vi "interfaz para quiz1 (1).vi"() -> ()   [LabVIEW 2020]
panel:
  in  "stop":bool
  out "Led 3":bool
  out "Led 2":bool
  out "Led 1":bool
  in  "Pulsador 3":bool
  in  "Pulsador 2":bool
  in  "Pulsador 1":bool
  out "tiempo(ms)":i32=1000
  out "Contador":i32
  in  "Insertar trama":string
  out "RESPUESTA":string="\n      \n           "
  in  "Ingreso de comandos":string
  in  "?":bool
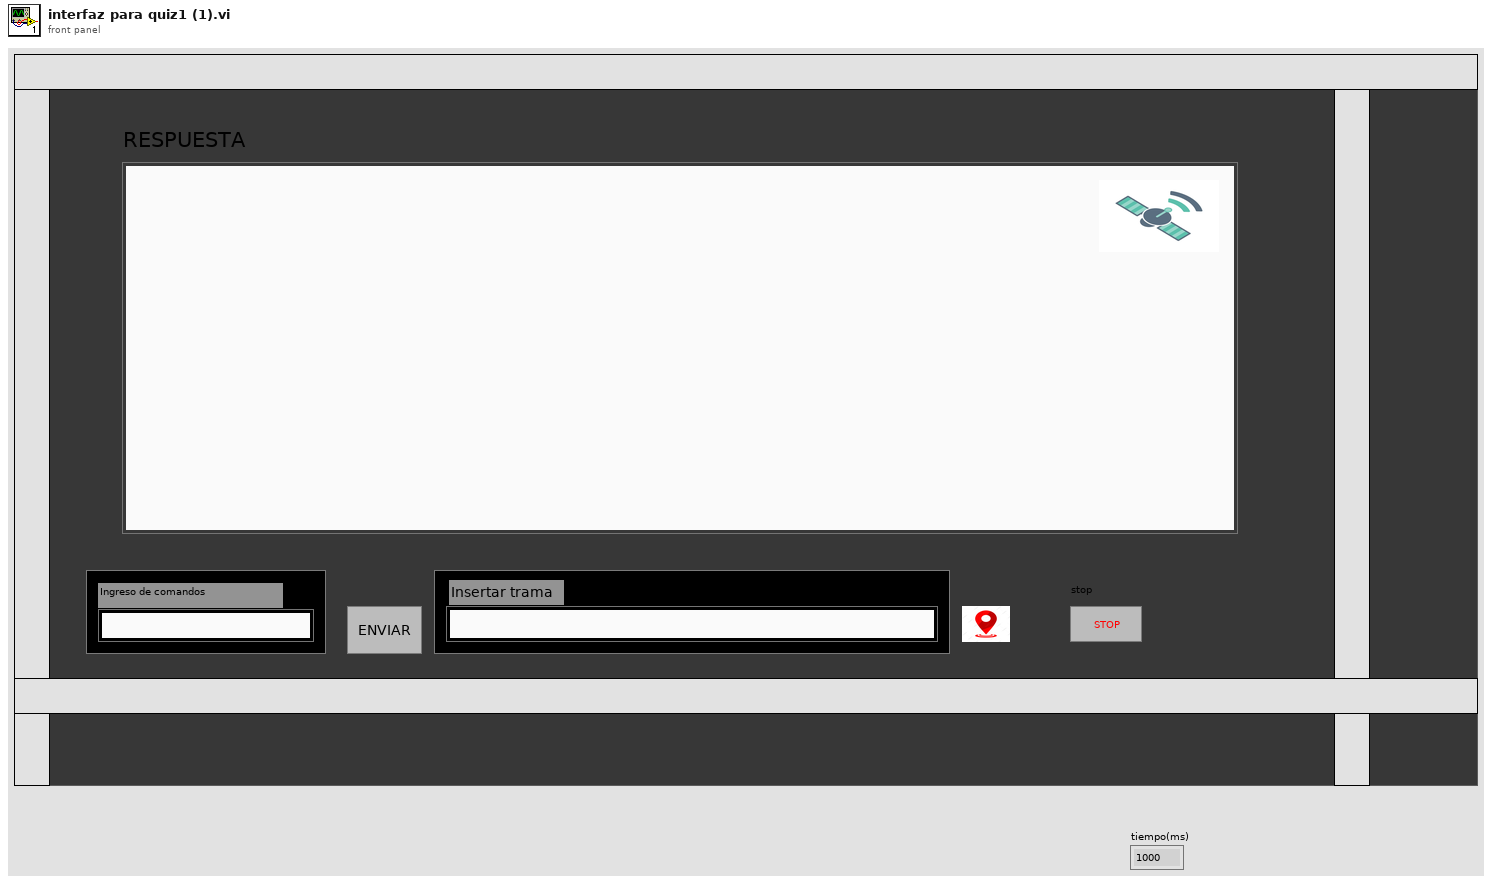
[diagram p1: front panel]
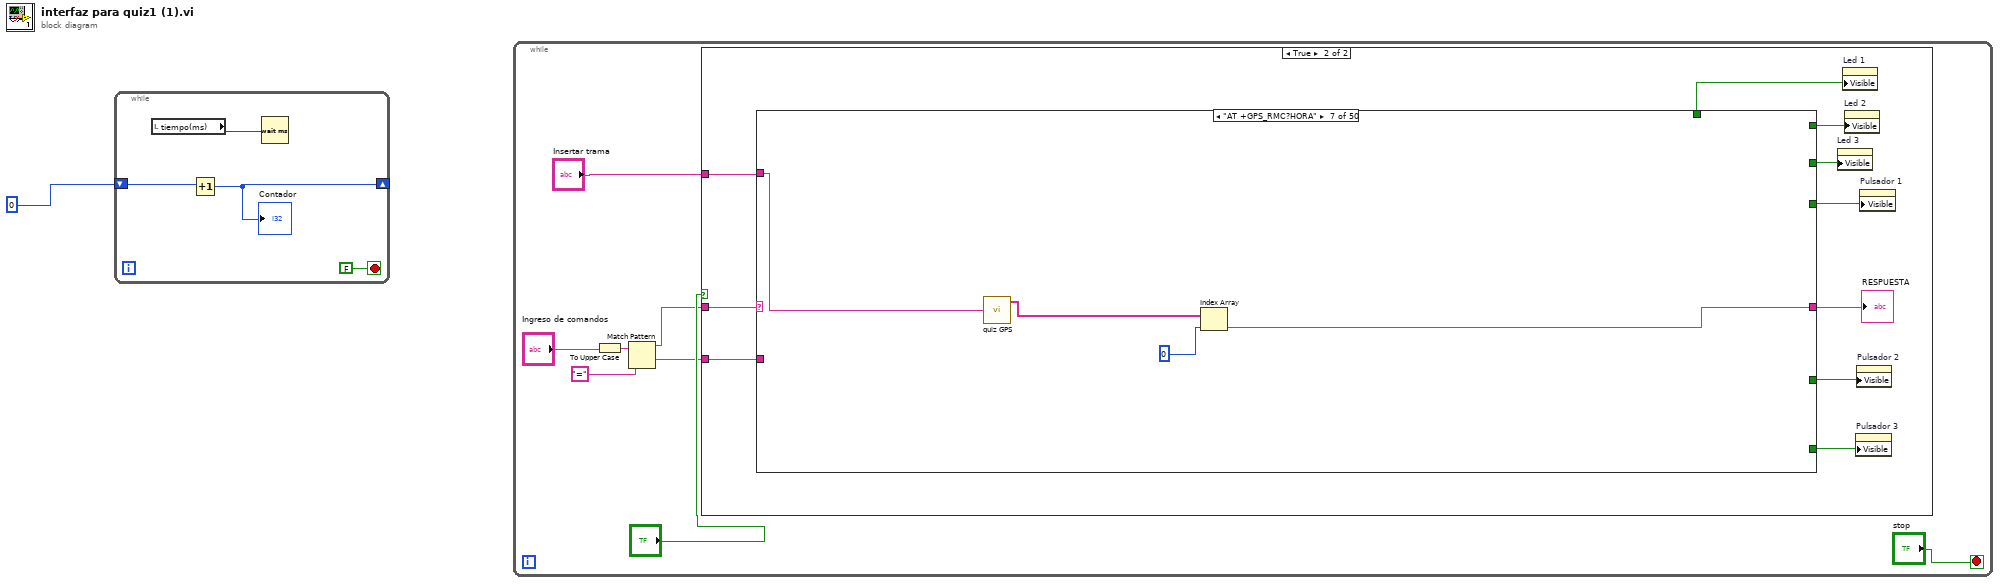
[diagram p0: block diagram]
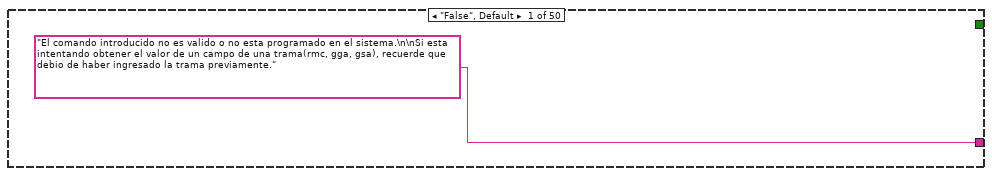
[diagram p3: hidden frame]
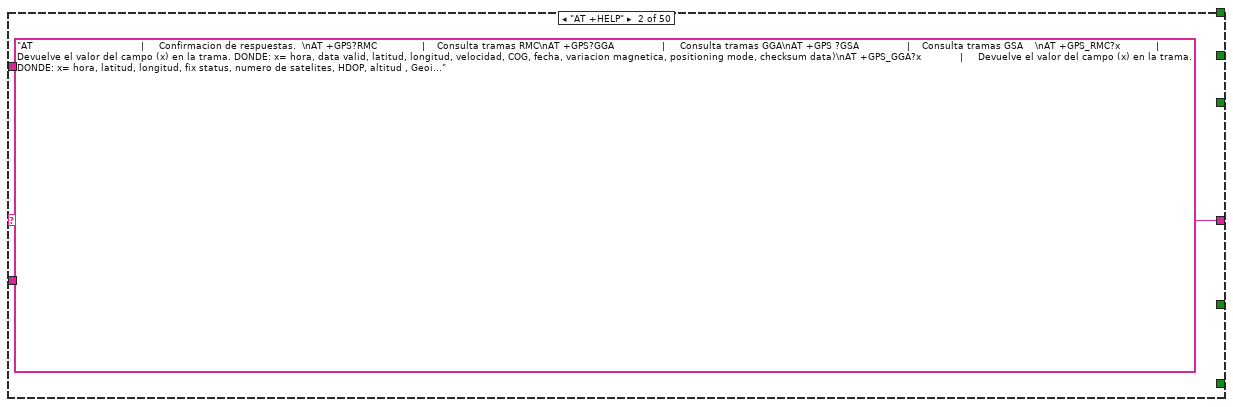
[diagram p4: hidden frame]
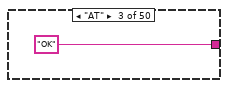
[diagram p5: hidden frame]
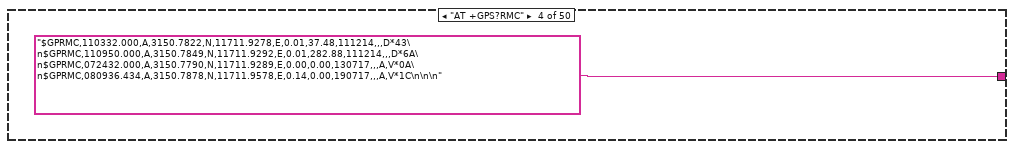
[diagram p6: hidden frame]
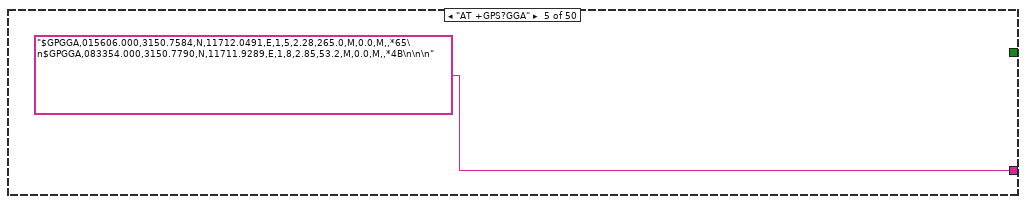
[diagram p7: hidden frame]
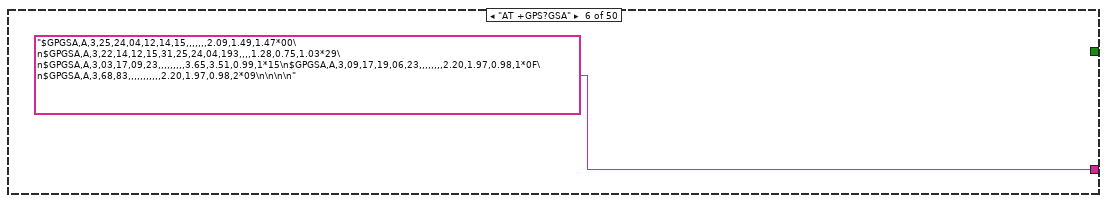
[diagram p8: hidden frame]
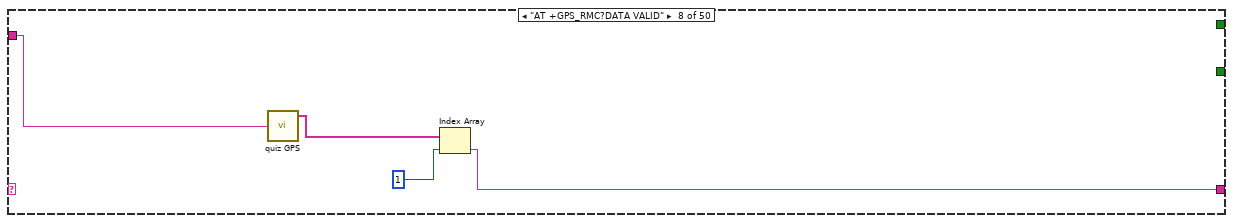
[diagram p9: hidden frame]
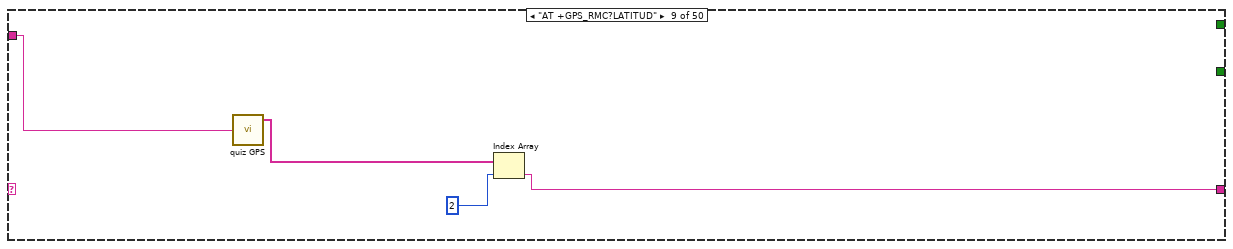
[diagram p10: hidden frame]
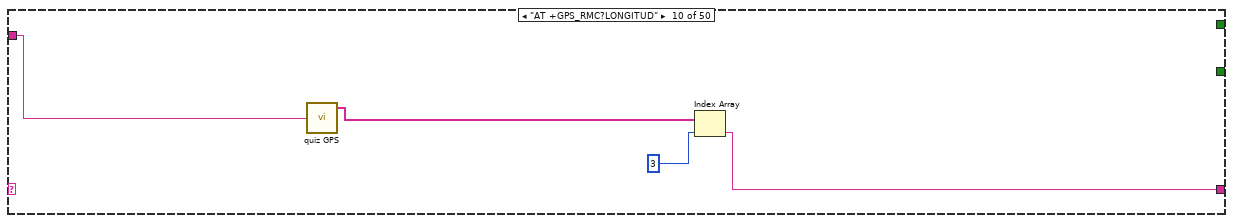
[diagram p11: hidden frame]
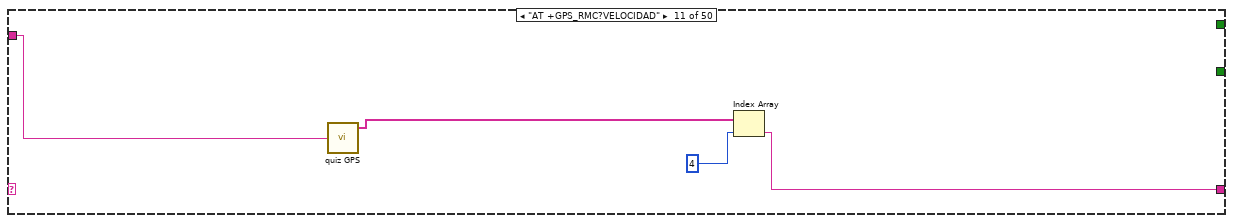
[diagram p12: hidden frame]
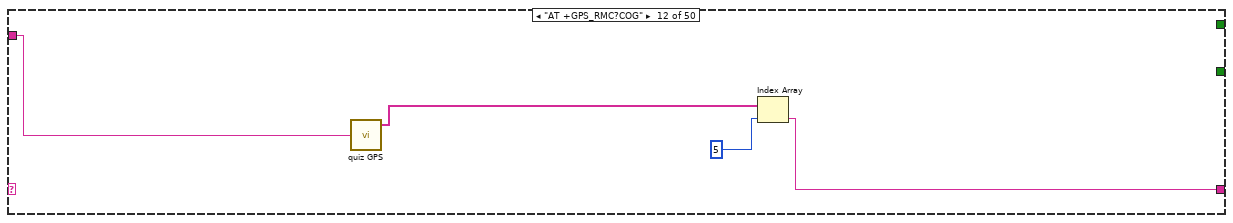
[diagram p13: hidden frame]
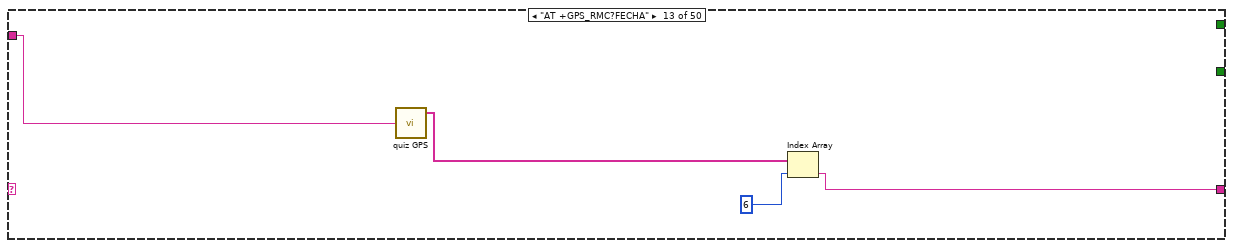
[diagram p14: hidden frame]
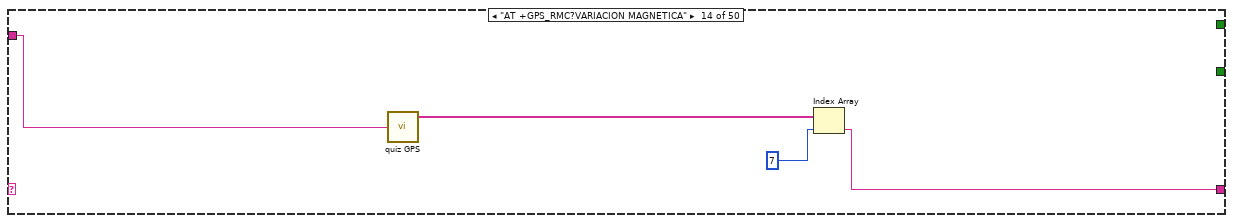
[diagram p15: hidden frame]
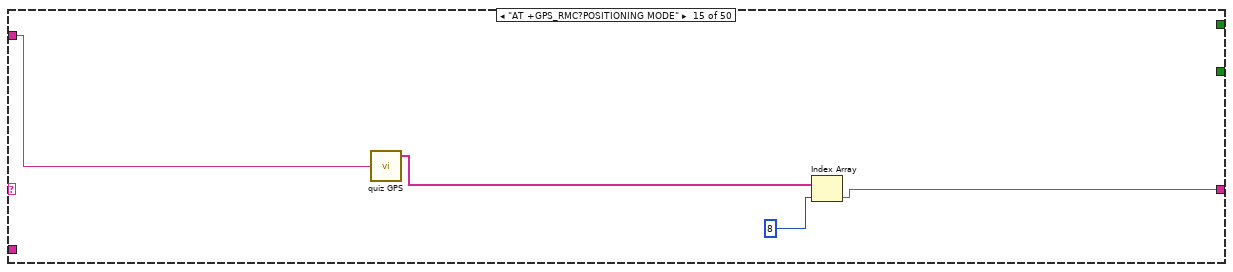
[diagram p16: hidden frame]
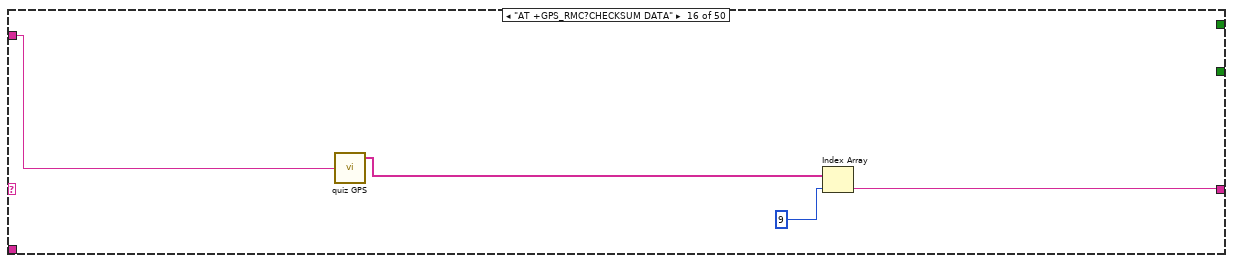
[diagram p17: hidden frame]
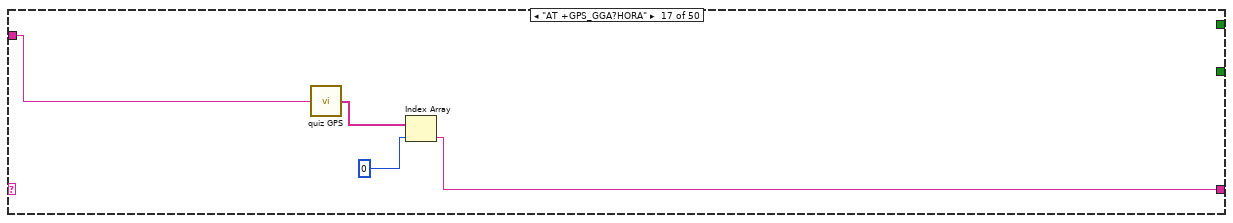
[diagram p18: hidden frame]
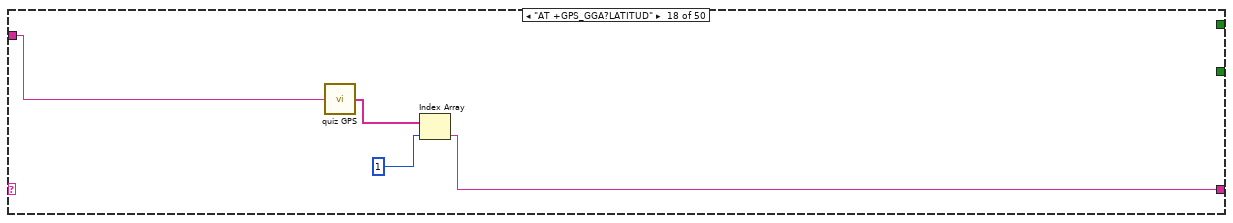
[diagram p19: hidden frame]
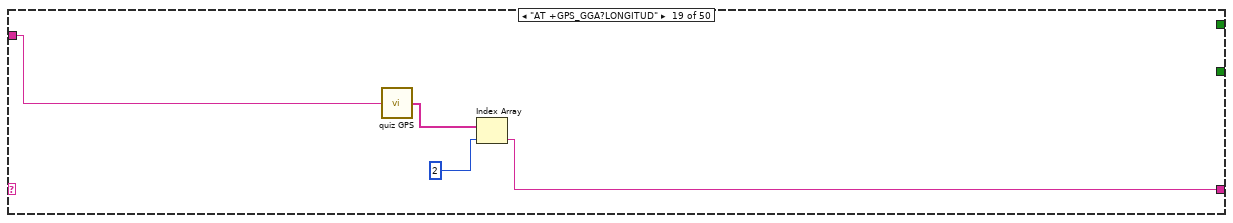
[diagram p20: hidden frame]
diagram:
  n1 = while {
    shift-right: [w2] -> _
    shift-left: 0 -> [w5]
    stop <- FALSE stop-if-true
    n2 = local read "tiempo(ms)"() -> (w3:i32)
    n3 = Increment(x=w5) -> (x+1=w2:i32)
    "Contador" <- w2
    n4 = Wait (ms)(milliseconds to wait=w3) -> ()  [unwired: 1 out]
  }
  n5 = while {
    stop <- "stop" stop-if-true
    n6 = To Upper Case(1:"Ingreso de comandos") -> (0:w10:string)
    n7 = Match Pattern(string=w10, regular expression="=") -> (before substring=w8:string, after substring=w7:string)  [unwired: 1 in, 2 out]
    n8 = case shown="True" "?" {
      tunnel: "Insertar trama" -> [_ w22]
      tunnel: w8 -> [_ w18]
      tunnel: w7 -> [_ w17]
      frame False {
      }
      frame True {
        n9 = case shown="\"AT +GPS_RMC?HORA\"" w18 {
          tunnel: ["El comando introducido no es valido o no esta programado en el sistema.\n\nSi esta intentando obtener el valor de un campo de una trama(rmc, gga, gsa), recuerde que debio de haber ingresado la trama previamente." "AT                                    |     Confirmacion de respuestas.  \nAT +GPS?RMC               |    Consulta tramas RMC\nAT +GPS?GGA                |     Consulta tramas GGA\nAT +GPS ?GSA                |    Consulta tramas GSA    \nAT +GPS_RMC?x            |     Devuelve el valor del campo (x) en la trama. DONDE: x= hora, data valid, latitud, longitud, velocidad, COG, fecha, variacion magnetica, positioning mode, checksum data)\nAT +GPS_GGA?x             |     Devuelve el valor del campo (x) en la trama. DONDE: x= hora, latitud, longitud, fix status, numero de satelites, HDOP, altitud , Geoid Separation, DGPS AGE, DGPS, ID checksum data)\nAT +GPS_GSA?x              |     Devuelve el valor del campo (x) en la trama. DONDE: x= mode, fix status, su1, su2, su3, su4, su5, su6, su7, su8 ,su9, su10, su11, su12, PDOP, HDOP, VDOP, checksum data )      y     su: satellite usado\nAT +TIMEPC                     |     Consulta la hora actual de tu pc.\nAT +CAMBIARTIEMPO=t |  Cambia cada cuanto tiempo aumenta la variable contador.                   DONDE:   t = lapzo de tiempo en (milisegundos) que desea que deba transcurrir para el aumento del contador.\nAT +LEERCONTADOR         | Lee la variable contador.                                                                              \nAT +LEERLEDS                   |  Lee estado de los led.                                                                       \nAT+MODIFICARLEDS      | Modifica el estado de los pulsadores de los leds.\n\n      \n           " "OK" "$GPRMC,110332.000,A,3150.7822,N,11711.9278,E,0.01,37.48,111214,,,D*43\n$GPRMC,110950.000,A,3150.7849,N,11711.9292,E,0.01,282.88,111214,,,D*6A\n$GPRMC,072432.000,A,3150.7790,N,11711.9289,E,0.00,0.00,130717,,,A,V*0A\n$GPRMC,080936.434,A,3150.7878,N,11711.9578,E,0.14,0.00,190717,,,A,V*1C\n\n\n" "$GPGGA,015606.000,3150.7584,N,11712.0491,E,1,5,2.28,265.0,M,0.0,M,,*65\n$GPGGA,083354.000,3150.7790,N,11711.9289,E,1,8,2.85,53.2,M,0.0,M,,*4B\n\n\n" "$GPGSA,A,3,25,24,04,12,14,15,,,,,,,2.09,1.49,1.47*00\n$GPGSA,A,3,22,14,12,15,31,25,24,04,193,,,,1.28,0.75,1.03*29\n$GPGSA,A,3,03,17,09,23,,,,,,,,,3.65,3.51,0.99,1*15\n$GPGSA,A,3,09,17,19,06,23,,,,,,,,2.20,1.97,0.98,1*0F\n$GPGSA,A,3,68,83,,,,,,,,,,,2.20,1.97,0.98,2*09\n\n\n\n" w32 w34 w38 w42 w46 w50 w54 w58 w62 w66 w70 w74 w78 w82 w86 w90 w94 w98 w102 w106 w110 w114 w118 w122 w126 w130 w134 w138 w142 w146 w150 w154 w158 w162 w166 w170 w174 w178 w182 w187 w197 w200 _ _] -> w23
          tunnel: w22 -> [_ _ _ _ _ _ w30 w36 w40 w44 w48 w52 w56 w60 w64 w68 w73 w75 w79 w83 w87 w91 w95 w99 w103 w107 w111 w115 w119 w123 w127 w131 w135 w139 w143 w147 w151 w155 w159 w163 w167 w171 w175 w179 w183 _ _ _ _ _]
          tunnel: [_ _ _ _ _ _ _ _ _ _ _ _ _ _ _ _ _ _ _ _ _ _ _ _ _ _ _ _ _ _ _ _ _ _ _ _ _ _ _ _ _ _ _ _ _ _ _ _ _ w208] -> w21
          tunnel: [_ _ _ _ _ _ _ _ _ _ _ _ _ _ _ _ _ _ _ _ _ _ _ _ _ _ _ _ _ _ _ _ _ _ _ _ _ _ _ _ _ _ _ _ _ _ _ _ _ w208] -> w20
          tunnel: [_ _ _ _ _ _ _ _ _ _ _ _ _ _ _ _ _ _ _ _ _ _ _ _ _ _ _ _ _ _ _ _ _ _ _ _ _ _ _ _ _ _ _ _ _ _ _ _ _ w208] -> w19
          tunnel: w17 -> [_ _ _ _ _ _ _ _ _ _ _ _ _ _ _ _ _ _ _ _ _ _ _ _ _ _ _ _ _ _ _ _ _ _ _ _ _ _ _ _ _ _ _ _ _ _ w199 _ _ _]
          tunnel: [_ _ _ _ _ _ _ _ _ _ _ _ _ _ _ _ _ _ _ _ _ _ _ _ _ _ _ _ _ _ _ _ _ _ _ _ _ _ _ _ _ _ _ _ _ _ _ _ w204 _] -> w16
          tunnel: [_ _ _ _ _ _ _ _ _ _ _ _ _ _ _ _ _ _ _ _ _ _ _ _ _ _ _ _ _ _ _ _ _ _ _ _ _ _ _ _ _ _ _ _ _ _ _ _ w204 _] -> w15
          tunnel: [_ _ _ _ _ _ _ _ _ _ _ _ _ _ _ _ _ _ _ _ _ _ _ _ _ _ _ _ _ _ _ _ _ _ _ _ _ _ _ _ _ _ _ _ _ _ _ _ w204 _] -> w14
          frame "False", Default {
          }
          frame "AT +HELP" {
          }
          frame "AT" {
          }
          frame "AT +GPS?RMC" {
          }
          frame "AT +GPS?GGA" {
          }
          frame "AT +GPS?GSA" {
          }
          frame "AT +GPS_RMC?HORA" {
            n10 = call "quiz GPS.vi"("TRAMA"=w30) -> ("Arreglo salida RMC"=w31:string[])  [unwired: 2 out]
            n11 = Index Array(array=w31, index=0) -> (element=w32:string)
          }
          frame "AT +GPS_RMC?DATA VALID" {
            n12 = call "quiz GPS.vi"("TRAMA"=w36) -> ("Arreglo salida RMC"=w35:string[])  [unwired: 2 out]
            n13 = Index Array(array=w35, index=1) -> (element=w34:string)
          }
          frame "AT +GPS_RMC?LATITUD" {
            n14 = call "quiz GPS.vi"("TRAMA"=w40) -> ("Arreglo salida RMC"=w39:string[])  [unwired: 2 out]
            n15 = Index Array(array=w39, index=2) -> (element=w38:string)
          }
          frame "AT +GPS_RMC?LONGITUD" {
            n16 = call "quiz GPS.vi"("TRAMA"=w44) -> ("Arreglo salida RMC"=w43:string[])  [unwired: 2 out]
            n17 = Index Array(array=w43, index=3) -> (element=w42:string)
          }
          frame "AT +GPS_RMC?VELOCIDAD" {
            n18 = call "quiz GPS.vi"("TRAMA"=w48) -> ("Arreglo salida RMC"=w47:string[])  [unwired: 2 out]
            n19 = Index Array(array=w47, index=4) -> (element=w46:string)
          }
          frame "AT +GPS_RMC?COG" {
            n20 = call "quiz GPS.vi"("TRAMA"=w52) -> ("Arreglo salida RMC"=w51:string[])  [unwired: 2 out]
            n21 = Index Array(array=w51, index=5) -> (element=w50:string)
          }
          frame "AT +GPS_RMC?FECHA" {
            n22 = call "quiz GPS.vi"("TRAMA"=w56) -> ("Arreglo salida RMC"=w55:string[])  [unwired: 2 out]
            n23 = Index Array(array=w55, index=6) -> (element=w54:string)
          }
          frame "AT +GPS_RMC?VARIACION MAGNETICA" {
            n24 = call "quiz GPS.vi"("TRAMA"=w60) -> ("Arreglo salida RMC"=w59:string[])  [unwired: 2 out]
            n25 = Index Array(array=w59, index=7) -> (element=w58:string)
          }
          frame "AT +GPS_RMC?POSITIONING MODE" {
            n26 = call "quiz GPS.vi"("TRAMA"=w64) -> ("Arreglo salida RMC"=w63:string[])  [unwired: 2 out]
            n27 = Index Array(array=w63, index=8) -> (element=w62:string)
          }
          frame "AT +GPS_RMC?CHECKSUM DATA" {
            n28 = call "quiz GPS.vi"("TRAMA"=w68) -> ("Arreglo salida RMC"=w67:string[])  [unwired: 2 out]
            n29 = Index Array(array=w67, index=9) -> (element=w66:string)
          }
          frame "AT +GPS_GGA?HORA" {
            n30 = call "quiz GPS.vi"("TRAMA"=w73) -> ("Arreglo salida GGA"=w71:string[])  [unwired: 2 out]
            n31 = Index Array(array=w71, index=0) -> (element=w70:string)
          }
          frame "AT +GPS_GGA?LATITUD" {
            n32 = call "quiz GPS.vi"("TRAMA"=w75) -> ("Arreglo salida GGA"=w76:string[])  [unwired: 2 out]
            n33 = Index Array(array=w76, index=1) -> (element=w74:string)
          }
          frame "AT +GPS_GGA?LONGITUD" {
            n34 = call "quiz GPS.vi"("TRAMA"=w79) -> ("Arreglo salida GGA"=w80:string[])  [unwired: 2 out]
            n35 = Index Array(array=w80, index=2) -> (element=w78:string)
          }
          frame "AT +GPS_GGA?FIX STATUS" {
            n36 = call "quiz GPS.vi"("TRAMA"=w83) -> ("Arreglo salida GGA"=w84:string[])  [unwired: 2 out]
            n37 = Index Array(array=w84, index=3) -> (element=w82:string)
          }
          frame "AT +GPS_GGA?NUMERO DE SATELITES" {
            n38 = call "quiz GPS.vi"("TRAMA"=w87) -> ("Arreglo salida GGA"=w88:string[])  [unwired: 2 out]
            n39 = Index Array(array=w88, index=4) -> (element=w86:string)
          }
          frame "AT +GPS_GGA?HDOP" {
            n40 = call "quiz GPS.vi"("TRAMA"=w91) -> ("Arreglo salida GGA"=w92:string[])  [unwired: 2 out]
            n41 = Index Array(array=w92, index=5) -> (element=w90:string)
          }
          frame "AT +GPS_GGA?ALTITUD" {
            n42 = call "quiz GPS.vi"("TRAMA"=w95) -> ("Arreglo salida GGA"=w96:string[])  [unwired: 2 out]
            n43 = Index Array(array=w96, index=6) -> (element=w94:string)
          }
          frame "AT +GPS_GGA?GEOID SEPARATION" {
            n44 = call "quiz GPS.vi"("TRAMA"=w99) -> ("Arreglo salida GGA"=w100:string[])  [unwired: 2 out]
            n45 = Index Array(array=w100, index=7) -> (element=w98:string)
          }
          frame "AT +GPS_GGA?DGPS AGE" {
            n46 = call "quiz GPS.vi"("TRAMA"=w103) -> ("Arreglo salida GGA"=w104:string[])  [unwired: 2 out]
            n47 = Index Array(array=w104, index=8) -> (element=w102:string)
          }
          frame "AT +GPS_GGA?DGPS ID" {
            n48 = call "quiz GPS.vi"("TRAMA"=w107) -> ("Arreglo salida GGA"=w108:string[])  [unwired: 2 out]
            n49 = Index Array(array=w108, index=9) -> (element=w106:string)
          }
          frame "AT +GPS_GGA?CHECKSUM DATA" {
            n50 = call "quiz GPS.vi"("TRAMA"=w111) -> ("Arreglo salida GGA"=w112:string[])  [unwired: 2 out]
            n51 = Index Array(array=w112, index=10) -> (element=w110:string)
          }
          frame "AT +GPS_GSA?MODE" {
            n52 = call "quiz GPS.vi"("TRAMA"=w115) -> ("Arreglo salida GSA"=w116:string[])  [unwired: 2 out]
            n53 = Index Array(array=w116, index=0) -> (element=w114:string)
          }
          frame "AT +GPS_GSA?FIX STATUS" {
            n54 = call "quiz GPS.vi"("TRAMA"=w119) -> ("Arreglo salida GSA"=w120:string[])  [unwired: 2 out]
            n55 = Index Array(array=w120, index=1) -> (element=w118:string)
          }
          frame "AT +GPS_GSA?SU1" {
            n56 = call "quiz GPS.vi"("TRAMA"=w123) -> ("Arreglo salida GSA"=w124:string[])  [unwired: 2 out]
            n57 = Index Array(array=w124, index=2) -> (element=w122:string)
          }
          frame "AT +GPS_GSA?SU2" {
            n58 = call "quiz GPS.vi"("TRAMA"=w127) -> ("Arreglo salida GSA"=w128:string[])  [unwired: 2 out]
            n59 = Index Array(array=w128, index=3) -> (element=w126:string)
          }
          frame "AT +GPS_GSA?SU3" {
            n60 = call "quiz GPS.vi"("TRAMA"=w131) -> ("Arreglo salida GSA"=w132:string[])  [unwired: 2 out]
            n61 = Index Array(array=w132, index=4) -> (element=w130:string)
          }
          frame "AT +GPS_GSA?SU4" {
            n62 = call "quiz GPS.vi"("TRAMA"=w135) -> ("Arreglo salida GSA"=w136:string[])  [unwired: 2 out]
            n63 = Index Array(array=w136, index=5) -> (element=w134:string)
          }
          frame "AT +GPS_GSA?SU5" {
            n64 = call "quiz GPS.vi"("TRAMA"=w139) -> ("Arreglo salida GSA"=w140:string[])  [unwired: 2 out]
            n65 = Index Array(array=w140, index=6) -> (element=w138:string)
          }
          frame "AT +GPS_GSA?SU6" {
            n66 = call "quiz GPS.vi"("TRAMA"=w143) -> ("Arreglo salida GSA"=w144:string[])  [unwired: 2 out]
            n67 = Index Array(array=w144, index=7) -> (element=w142:string)
          }
          frame "AT +GPS_GSA?SU7" {
            n68 = call "quiz GPS.vi"("TRAMA"=w147) -> ("Arreglo salida GSA"=w148:string[])  [unwired: 2 out]
            n69 = Index Array(array=w148, index=8) -> (element=w146:string)
          }
          frame "AT +GPS_GSA?SU8" {
            n70 = call "quiz GPS.vi"("TRAMA"=w151) -> ("Arreglo salida GSA"=w152:string[])  [unwired: 2 out]
            n71 = Index Array(array=w152, index=9) -> (element=w150:string)
          }
          frame "AT +GPS_GSA?SU9" {
            n72 = call "quiz GPS.vi"("TRAMA"=w155) -> ("Arreglo salida GSA"=w156:string[])  [unwired: 2 out]
            n73 = Index Array(array=w156, index=10) -> (element=w154:string)
          }
          frame "AT +GPS_GSA?SU10" {
            n74 = call "quiz GPS.vi"("TRAMA"=w159) -> ("Arreglo salida GSA"=w160:string[])  [unwired: 2 out]
            n75 = Index Array(array=w160, index=11) -> (element=w158:string)
          }
          frame "AT +GPS_GSA?SU11" {
            n76 = call "quiz GPS.vi"("TRAMA"=w163) -> ("Arreglo salida GSA"=w164:string[])  [unwired: 2 out]
            n77 = Index Array(array=w164, index=12) -> (element=w162:string)
          }
          frame "AT +GPS_GSA?SU12" {
            n78 = call "quiz GPS.vi"("TRAMA"=w167) -> ("Arreglo salida GSA"=w168:string[])  [unwired: 2 out]
            n79 = Index Array(array=w168, index=13) -> (element=w166:string)
          }
          frame "AT +GPS_GSA?PDOP" {
            n80 = call "quiz GPS.vi"("TRAMA"=w171) -> ("Arreglo salida GSA"=w172:string[])  [unwired: 2 out]
            n81 = Index Array(array=w172, index=14) -> (element=w170:string)
          }
          frame "AT +GPS_GSA?HDOP" {
            n82 = call "quiz GPS.vi"("TRAMA"=w175) -> ("Arreglo salida GSA"=w176:string[])  [unwired: 2 out]
            n83 = Index Array(array=w176, index=15) -> (element=w174:string)
          }
          frame "AT +GPS_GSA?VDOP" {
            n84 = call "quiz GPS.vi"("TRAMA"=w179) -> ("Arreglo salida GSA"=w180:string[])  [unwired: 2 out]
            n85 = Index Array(array=w180, index=16) -> (element=w178:string)
          }
          frame "AT +GPS_GSA?CHECKSUM DATA" {
            n86 = call "quiz GPS.vi"("TRAMA"=w183) -> ("Arreglo salida GSA"=w184:string[])  [unwired: 2 out]
            n87 = Index Array(array=w184, index=17) -> (element=w182:string)
          }
          frame "AT +TIMEPC" {
            n88 = Get Date/Time String() -> (date string=w192:string, time string=w190:string)  [unwired: 3 in]
            n89 = Concatenate Strings("Fecha: " ("string"), w192) -> (w189:string)
            n90 = Concatenate Strings("Hora: " ("string"), w190) -> (w188:string)
            n91 = Concatenate Strings(w189, "\r\n", w188) -> (w187:string)
          }
          frame "AT +CAMBIARTIEMPO" {
            n92 = Decimal String To Number(string=w199) -> (number=w198:i32)  [unwired: 2 in, 1 out]
            "tiempo(ms)" <- w198
            n93 = Number To Decimal String(number=w198) -> (decimal integer string=w195:string)  [unwired: 1 in]
            n94 = Concatenate Strings("El tiempo ha sido modificado. visualice en el indicador de abajo llamado tiempo(ms).\n\nEl nuevo tiempo indicado es:       ", w195, "    milisegundos") -> (w197:string)
          }
          frame "AT +LEERCONTADOR" {
            n95 = local read "Contador"() -> (w203:i32)
            n96 = Number To Decimal String(number=w203) -> (decimal integer string=w201:string)  [unwired: 1 in]
            n97 = Concatenate Strings("El valor actual del contador es:    " ("string"), w201) -> (w200:string)
          }
          frame "AT +LEERLEDS" {
            w204 = TRUE
            n98 = local read "Pulsador 3"() -> (→"Led 3":bool)
            n99 = local read "Pulsador 1"() -> (→"Led 1":bool)
            n100 = local read "Pulsador 2"() -> (→"Led 2":bool)
          }
          frame "AT +MODIFICARLEDS" {
            w208 = TRUE
          }
        }
        "RESPUESTA" <- w23
        n101 = property on="Led 3" class="Bool (strict)"("Visible"=w14) -> ()  [unwired: 2 in, 2 out]
        n102 = property on="Led 1" class="Bool (strict)"("Visible"=w16) -> ()  [unwired: 2 in, 2 out]
        n103 = property on="Led 2" class="Bool (strict)"("Visible"=w15) -> ()  [unwired: 2 in, 2 out]
        n104 = property on="Pulsador 3" class="Bool (strict)"("Visible"=w19) -> ()  [unwired: 2 in, 2 out]
        n105 = property on="Pulsador 2" class="Bool (strict)"("Visible"=w20) -> ()  [unwired: 2 in, 2 out]
        n106 = property on="Pulsador 1" class="Bool (strict)"("Visible"=w21) -> ()  [unwired: 2 in, 2 out]
      }
    }
  }
